vi "getTimeStamps.vi"(8 "error in (no error)":errorcluster, 11 "ScriptEventList in":refnum<class "ScriptEventList.lvclass">) -> (0 "error out":errorcluster, 2 "timeStamps (s)":dbl[](array[numeric]), 3 "ScriptEventList out":refnum<class "ScriptEventList.lvclass">)   [LabVIEW 2009, in "Tools.lvlib" / "Scripting.lvlib" / "ScriptEventList.lvclass"]
uses:
  ScriptEventList.lvclass
  ScriptEventList.lvclass/ScriptEventList.ctl
  ScriptEvent.lvclass
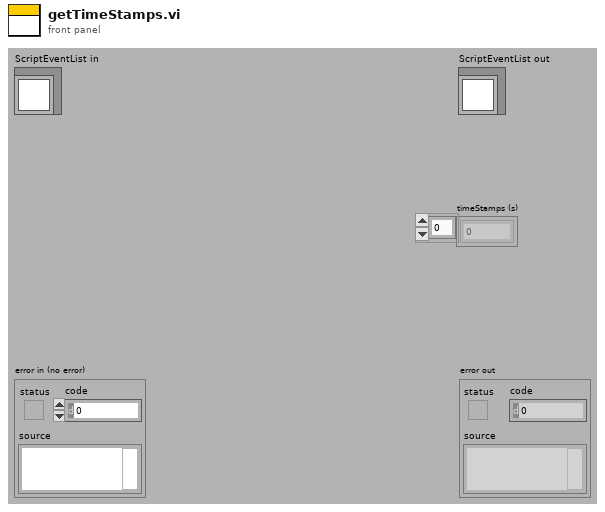
[diagram p1: front panel]
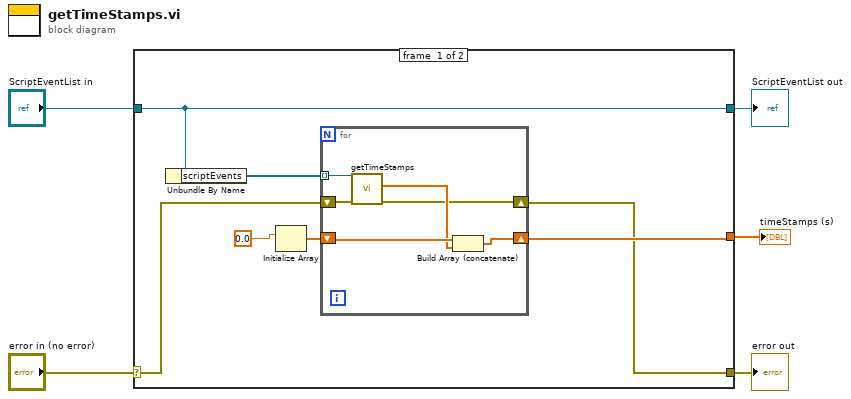
[diagram p0: block diagram]
diagram:
  n1 = case shown="No Error" "error in (no error)" {
    selector: "error in (no error)" -> [w7 w20]
    tunnel: [w6 w20] -> w4
    tunnel: [w12 w19] -> w2
    tunnel: "ScriptEventList in" -> [w12 w19]
    tunnel: [w8 _] -> w1
    frame #0 {
      n2 = Unbundle By Name(w12) -> ("scriptEvents"=w11:refnum<class "ScriptEvent.lvclass">[])
      n3 = Initialize Array(0.0) -> (w9:dbl[])  [unwired: 1 in]
      n4 = for {
        tunnel: w11 -> [w18] mode=indexing
        shift-right: [w15] -> w8
        shift-left: w9 -> [w17]
        shift-right: [w13] -> w6
        shift-left: w7 -> [w14]
        n5 = call-dynamic "getTimeStamps.vi"("error in (no error)"=w14, "ScriptEvent in"=w18) -> ("error out"=w13:errorcluster, "timeStamps"=w16:dbl[])  [unwired: 7 in, 1 out]
        n6 = Build Array (concatenate)(w17, w16) -> (w15:dbl[])
      }
    }
    frame #1 {
    }
  }
  "error out" <- w4
  "ScriptEventList out" <- w2
  "timeStamps (s)" <- w1
